vi "Power-On Status.vi"(0 "VISA resource name":refnum<visa-resource-name>, 5 "Power On Status Clear (0 = Load Previous Enable Registers)":u16(ring) items=["Load Previous Enable Registers", "Clear Enable Registers"], 11 "error in (no error)":errorcluster) -> (4 "VISA resource name out":refnum<visa-resource-name>, 15 "error out":errorcluster)   [LabVIEW 2016, in "APT 300XAC Series.lvlib"]
doc: "Sets the power-on status clear bit. When set to 1 the Standard Event Enable register and Status Byte Enable registers will be cleared when power is turned ON. 0 setting indicates the Enable registers will be loaded with Enable register masks from non-volatile memory at power ON."
uses:
  APT 300XAC Series.lvlib
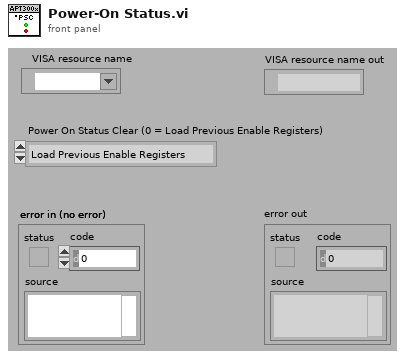
[diagram p1: front panel]
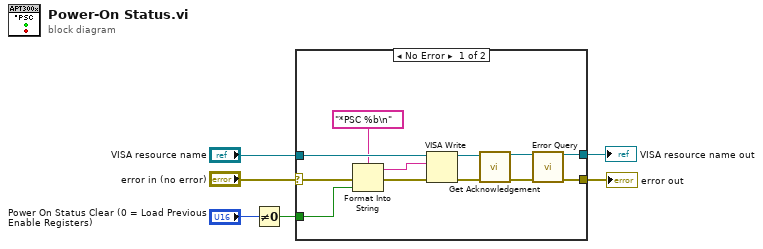
[diagram p0: block diagram]
diagram:
  n1 = Not Equal To 0?(x="Power On Status Clear (0 = Load Previous Enable Registers)") -> (x != 0?=w1:bool)
  n2 = case shown="No Error" "error in (no error)" {
    selector: "error in (no error)" -> [w12 w19]
    tunnel: [w18 w20] -> w4
    tunnel: [w17 w19] -> w3
    tunnel: "VISA resource name" -> [w16 w20]
    tunnel: w1 -> [w14 _]
    frame No Error {
      n3 = Format Into String(format string="*PSC %b\n" ("Command to Send (empty)"), error in=w12, w14) -> (resulting string=w13:string, error out=w11:errorcluster)  [unwired: 1 in]
      n4 = VISA Write(VISA resource name=w16, write buffer=w13, error in (no error)=w11) -> (VISA resource name out=w7:refnum<visa-resource-name>, error out=w8:errorcluster)  [unwired: 1 out]
      n5 = call "Get Acknowledgement.vi"("VISA resource name"=w7, "error in (no error)"=w8) -> ("VISA resource name out"=w10:refnum<visa-resource-name>, "error out"=w9:errorcluster)  [unwired: 12 in]
      n6 = call "Error Query.vi"("VISA resource name"=w10, "error in (no error)"=w9) -> ("VISA resource name out"=w18:refnum<visa-resource-name>, "error out"=w17:errorcluster)  [unwired: 10 in, 2 out]
    }
    frame Error {
    }
  }
  "VISA resource name out" <- w4
  "error out" <- w3
